vi "populate_multicolumn.vi"(6 "progress slider":refnum<vi>, 7 "selected item (index)":i32, 8 "error in (no error)":errorcluster, 10 "steps":T1[](array[typedef]), 11 "multicolumn list box":refnum<vi>) -> (0 "error out":errorcluster)   [LabVIEW 2010]
uses:
  common/clusters/plugin_specification.ctl
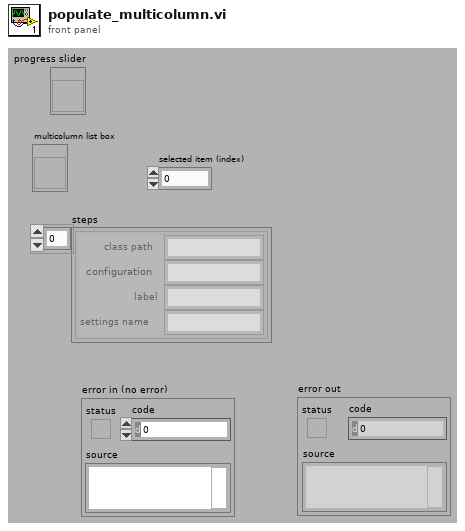
[diagram p1: front panel]
types:
  T1 = typedef "plugin_specification.ctl" = cluster{"class path":string, "configuration":string, "label":string, "settings name":string}
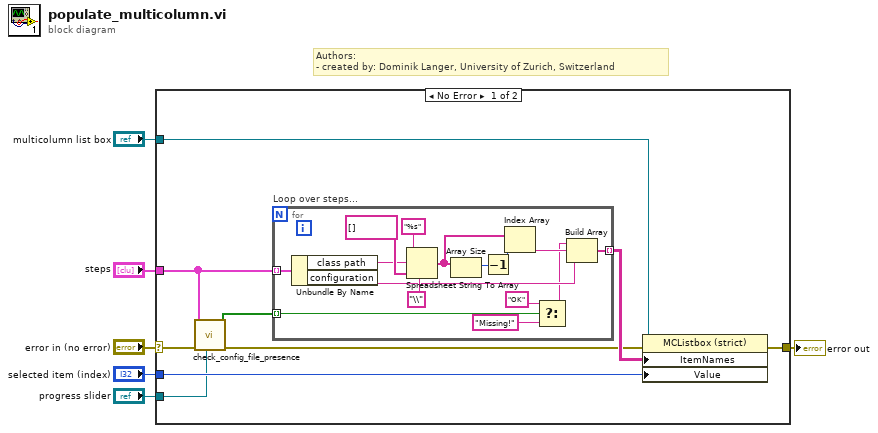
[diagram p0: block diagram]
diagram:
  # "Authors: \n- created by: Dominik Langer, University of Zurich, Switzerland"
  n1 = case shown="No Error" "error in (no error)" {
    selector: "error in (no error)" -> [w10 w30]
    tunnel: "steps" -> [w11 _]
    tunnel: [w9 w30] -> w2
    tunnel: "multicolumn list box" -> [w13 _]
    tunnel: "selected item (index)" -> [w14 _]
    tunnel: "progress slider" -> [w7 _]
    frame No Error {
      n2 = call "check_config_file_presence.vi"("progress slider"=w7, "error in (no error)"=w10, "steps"=w11) -> ("error out"=w9:errorcluster, "present?"=w8:bool[])  [unwired: 7 in]
      n3 = for "Loop over steps..." {
        tunnel: w11 -> [w29] mode=indexing
        tunnel: [w19] -> w12 mode=indexing
        tunnel: w8 -> [w18] mode=indexing
        n4 = Unbundle By Name(w29) -> ("class path"=w26:string, "configuration"=w21:string)
        n5 = Spreadsheet String To Array(delimiter (Tab)="\\" ("search string/char (-)"), format string="%s", spreadsheet string=w26, array type (2D Dbl)=string[] []) -> (array=w25:string[])
        n6 = Array Size(array=w25) -> (size(s)=w24:i32)
        n7 = Decrement(x=w24) -> (x-1=w23:i32)
        n8 = Index Array(array=w25, index=w23) -> (element=w20:string)
        n9 = Select(t="OK", s=w18, f="Missing!") -> (s? t:f=w17:string)
        n10 = Build Array(w17, w20, w21) -> (w19:string[])
      }
      n11 = property on="Property Node" class="MCListbox (strict)"(reference=w13, error in=w9, "ItemNames"=w12, "Value"=w14) -> ()  [unwired: 2 out]
    }
    frame Error {
    }
  }
  "error out" <- w2
